vi "Sensor Inputs.vi"(3 "error in":errorcluster) -> (0 "error out":errorcluster, 1 "data":bool[](array[boolean]), 2 "task out":refnum<k21>)   [LabVIEW 2014]
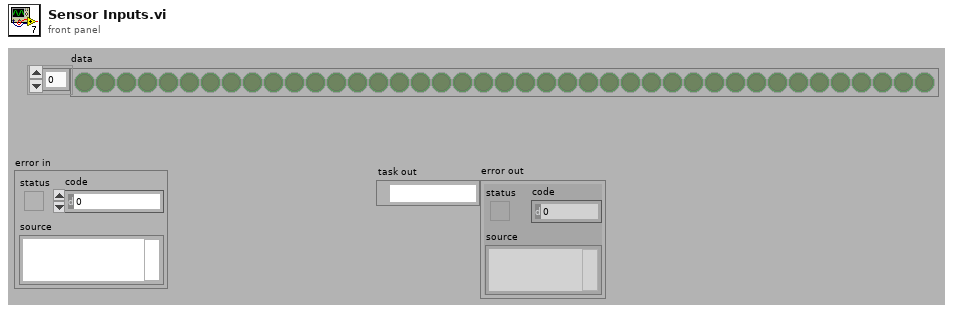
[diagram p1: front panel]
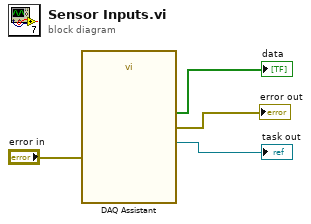
[diagram p0: block diagram]
diagram:
  n1 = call "DAQ Assistant"("error in"="error in") -> ("task out"=→"task out":refnum<k21>, "data"=→"data":bool[], "error out"=→"error out":errorcluster)  [unwired: 16 in]
